vi "lijnvolgen_al_dan_niet (SubVI).vi"(10 "OK Button":bool, 11 "ingelezen waardes reflectiesensor":dbl[](array[numeric])) -> (2 "Boolean":bool)   [LabVIEW 2019]
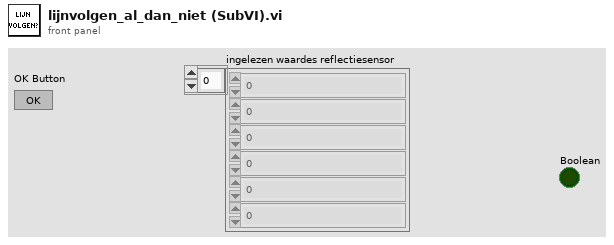
[diagram p1: front panel]
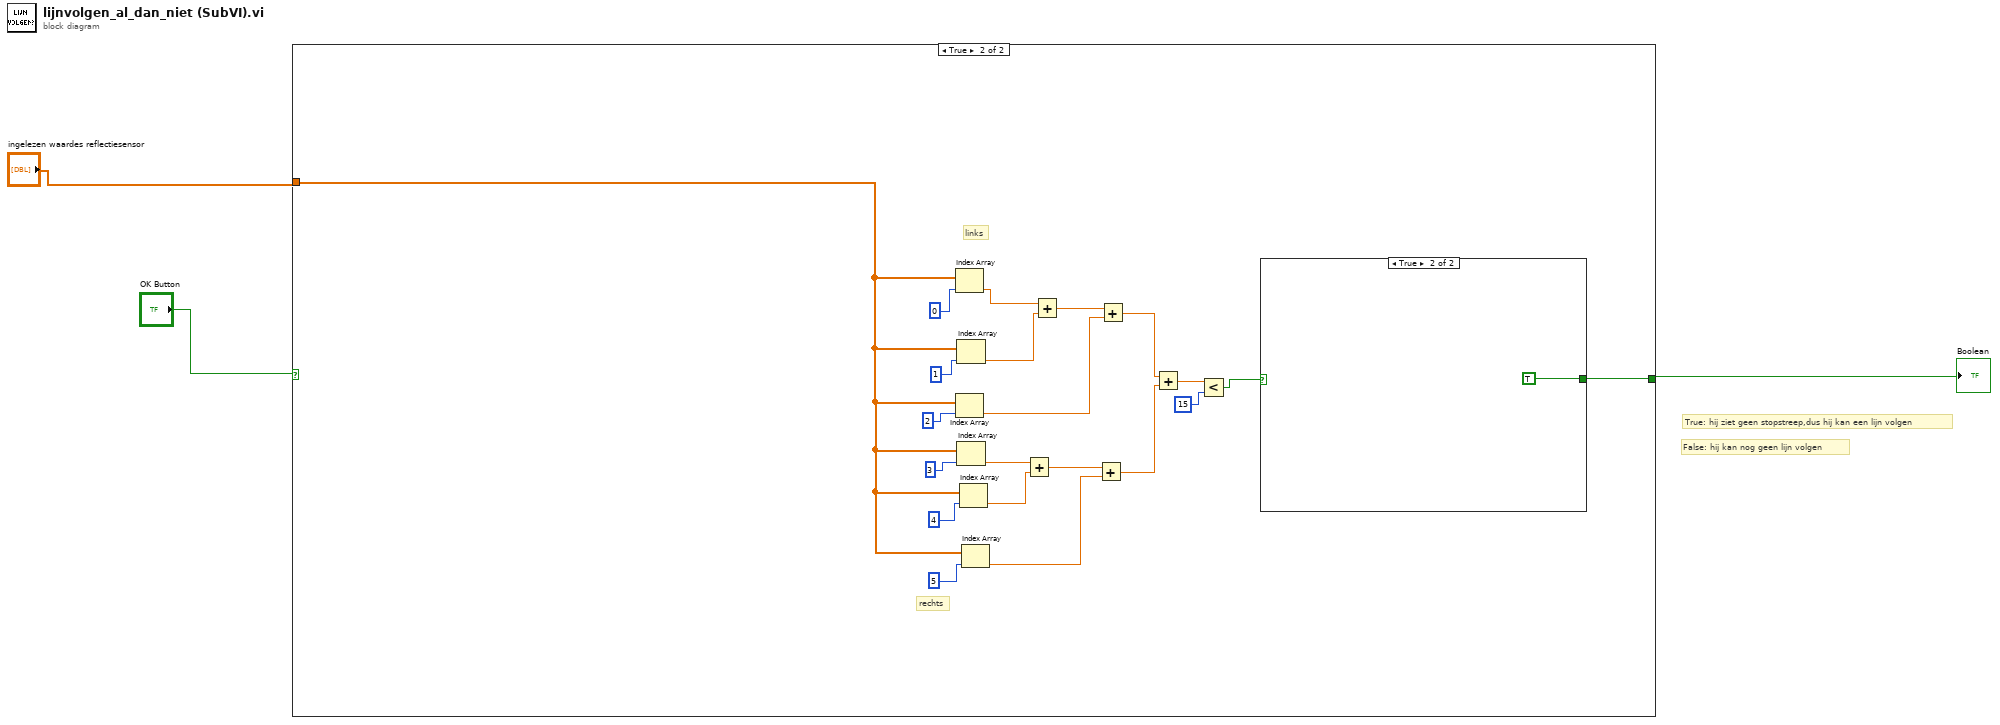
[diagram p0: block diagram]
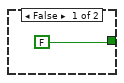
[diagram p2: hidden frame]
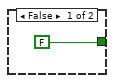
[diagram p3: hidden frame]
diagram:
  # "False: hij kan nog geen lijn volgen"
  # "True: hij ziet geen stopstreep,dus hij kan een lijn volgen"
  n1 = case shown="True" "OK Button" {
    tunnel: [FALSE w9] -> w1
    tunnel: "ingelezen waardes reflectiesensor" -> [_ w8]
    frame False {
    }
    frame True {
      # "links"
      # "rechts"
      n2 = Index Array(array=w8, index=0) -> (element=w16:dbl)
      n3 = Index Array(array=w8, index=2) -> (element=w19:dbl)
      n4 = Index Array(array=w8, index=1) -> (element=w17:dbl)
      n5 = Index Array(array=w8, index=3) -> (element=w20:dbl)
      n6 = Index Array(array=w8, index=4) -> (element=w21:dbl)
      n7 = Index Array(array=w8, index=5) -> (element=w22:dbl)
      n8 = Add(x=w20, y=w21) -> (x+y=w23:dbl)
      n9 = Add(x=w16, y=w17) -> (x+y=w18:dbl)
      n10 = Add(x=w23, y=w22) -> (x+y=w25:dbl)
      n11 = Add(x=w18, y=w19) -> (x+y=w24:dbl)
      n12 = Add(x=w24, y=w25) -> (x+y=w5:dbl)
      n13 = Less?(x=w5, y=15) -> (x < y?=w7:bool)
      n14 = case shown="True" w7 {
        tunnel: [FALSE TRUE] -> w9
        frame False {
        }
        frame True {
        }
      }
    }
  }
  "Boolean" <- w1
